vi "Project_Get all Build Spec Tags.vi"() -> ()   [LabVIEW 2019]
uses:
  ProjectBuilder.lvlib
panel:
  in  "Project Path":path
  in  "Build Specification Name":string
  in  "Target Name(\"\"> My Computer)":string
  out "Success?":bool
  out "Tag Values":variant[](array[variant])
  out "Tag Names":string[](array[string])
  out "error out":errorcluster
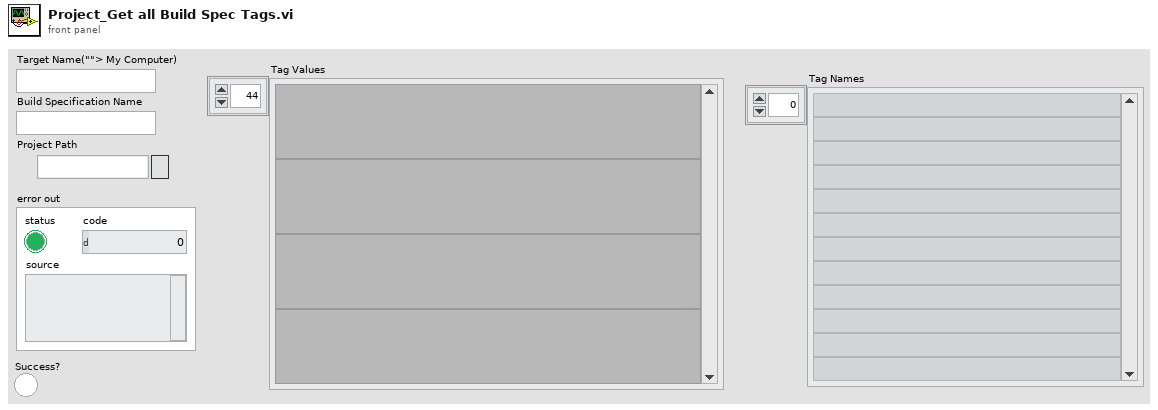
[diagram p1: front panel]
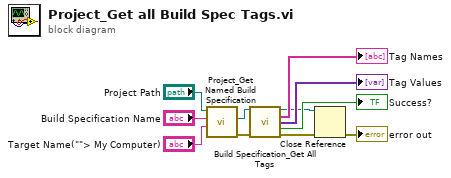
[diagram p0: block diagram]
diagram:
  n1 = call "Project_Get Named Build Specification.vi"("Target Name(\"\"> My Computer)"="Target Name(\"\"> My Computer)", "Build Specification Name"="Build Specification Name", "Project Path"="Project Path") -> ("error out"=w10:errorcluster, "Build Spec reference"=w11:refnum<vi>)  [unwired: 5 in, 2 out]
  n2 = call "Build Specification_Get All Tags.vi"("Build Spec reference in"=w11, "error in(no error)"=w10) -> ("Build Spec reference out"=w2:refnum<vi>, "Tag Names"=→"Tag Names":string[], "Tag Values"=→"Tag Values":variant[], "Success?"=→"Success?":bool, "error out"=w1:errorcluster)  [unwired: 9 in]
  n3 = Close Reference(reference=w2, error in (no error)=w1) -> (error out=→"error out":errorcluster)
